vi "Example - Time Profile Logger.vi"() -> ()   [LabVIEW 2016, in "SLL Debug.lvlib"]
uses:
  SLL Debug.lvlib
  _Typedefs/Time Profile Logger Command.ctl
panel:
  out "Profile Data[][]":string[][](array[string])
  out "Log Path":path
  # "Run this VI to see Time Profile Logger VI in action"
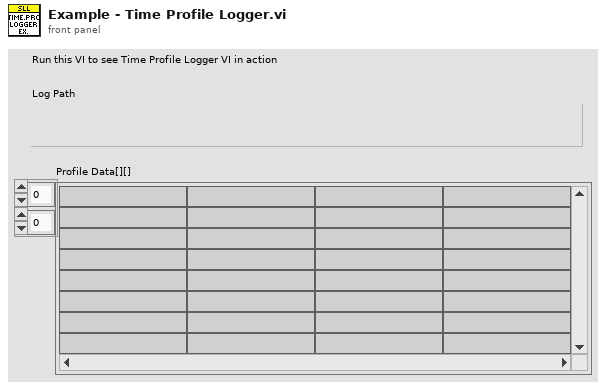
[diagram p1: front panel]
types:
  T1 = typedef "SLL Debug.lvlib/Time Profile Logger Command.ctl" = enum16{"Force Initialize", "Log", "Flush and Close"}
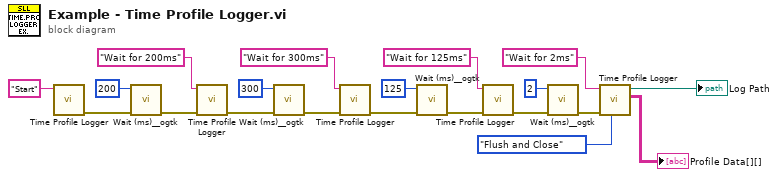
[diagram p0: block diagram]
diagram:
  n1 = call "Time Profile Logger.vi"("Primary Tag"="Start" ("Tag")) -> ("error out"=w20:errorcluster)  [unwired: 8 in, 2 out]
  n2 = call <userlib>:"Wait (ms)__ogtk.vi"("error in (no error)"=w20, "milliseconds to wait"=u32 200) -> ("error out"=w18:errorcluster)  [unwired: 8 in, 1 out]
  n3 = call "Time Profile Logger.vi"("error in (no error)"=w18, "Primary Tag"="Wait for 200ms" ("Tag")) -> ("error out"=w19:errorcluster)  [unwired: 7 in, 2 out]
  n4 = call <userlib>:"Wait (ms)__ogtk.vi"("error in (no error)"=w19, "milliseconds to wait"=u32 300) -> ("error out"=w14:errorcluster)  [unwired: 8 in, 1 out]
  n5 = call "Time Profile Logger.vi"("error in (no error)"=w14, "Primary Tag"="Wait for 300ms" ("Tag")) -> ("error out"=w15:errorcluster)  [unwired: 7 in, 2 out]
  n6 = call <userlib>:"Wait (ms)__ogtk.vi"("error in (no error)"=w15, "milliseconds to wait"=u32 125) -> ("error out"=w17:errorcluster)  [unwired: 8 in, 1 out]
  n7 = call "Time Profile Logger.vi"("error in (no error)"=w17, "Primary Tag"="Wait for 125ms" ("Tag")) -> ("error out"=w16:errorcluster)  [unwired: 7 in, 2 out]
  n8 = call <userlib>:"Wait (ms)__ogtk.vi"("error in (no error)"=w16, "milliseconds to wait"=u32 2) -> ("error out"=w8:errorcluster)  [unwired: 8 in, 1 out]
  n9 = call "Time Profile Logger.vi"("Command (Log)"=Time_Profile_Logger_Command."Flush and Close", "error in (no error)"=w8, "Primary Tag"="Wait for 2ms" ("Tag")) -> ("Profile Data[][]"=→"Profile Data[][]":string[][], "Log Path"=→"Log Path":path)  [unwired: 6 in, 1 out]
